vi "generate empty sample array.vi"(11 "file size":i32) -> (3 "output cluster":T1)   [LabVIEW 2014]
uses:
  Controls/Audio In.ctl
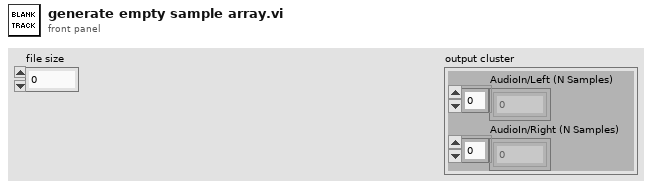
[diagram p1: front panel]
types:
  T1 = typedef "Audio In.ctl" = cluster{"AudioIn/Left (N Samples)":i16[], "AudioIn/Right (N Samples)":i16[]}
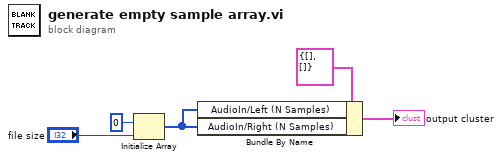
[diagram p0: block diagram]
diagram:
  n1 = Initialize Array(i16 0, "file size") -> (w4:i16[])
  n2 = Bundle By Name(cluster=T1 {"AudioIn/Left (N Samples)"=[], "AudioIn/Right (N Samples)"=[]} ("Track 3"), "AudioIn/Left (N Samples)"=w4, "AudioIn/Right (N Samples)"=w4) -> (→"output cluster":T1)
